vi "JPEG2000-Example.vi"() -> ()   [LabVIEW 2026]
uses:
  <vilib>/Utility/sysdir.llb/System Directory Type.ctl
panel:
  out "Image":T1(plugin-control)
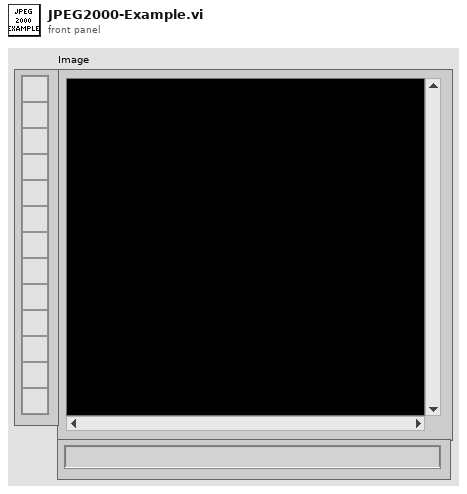
[diagram p1: front panel]
types:
  T1 = typedef "IMAQ Image.ctl" = refnum<image>
  T2 = typedef "System Directory Type.ctl" = i32
  T3 = typedef "Image Type" = u32
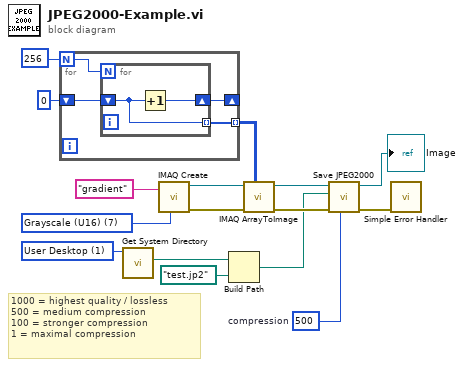
[diagram p0: block diagram]
diagram:
  w4 = T2 1 items=["User Home"=0, "User Desktop"=1, "User Documents"=2, "User Application Data"=3, "User Preferences"=4, "User Temporary"=5, "Public Documents"=6, "Public Application Data"=7, "Public Preferences"=8, "Public Cache"=13, "System Core Libraries"=9, "System Installed Libraries"=10, "Application Files"=11, "Boot Volume Root"=12] ("system directory type")
  w7 = 500  # compression
  w13 = T3 7 items=["Grayscale (U8)", "Grayscale (I16)", "Grayscale (SGL)", "Complex (CSG)", "RGB (U32)", "HSL (U32)", "RGB (U64)", "Grayscale (U16)"] ("Image Type")
  # "1000 = highest quality / lossless\n500 = medium compression\n100 = stronger compression\n1 = maximal compression"
  n1 = for {
    N: 256 -> [w20]
    shift-right: [w18] -> _
    shift-left: u16 0 -> [w19]
    tunnel: [w17] -> w11 mode=indexing
    n2 = for {
      N: w20 -> [_]
      shift-right: [w22] -> w18
      shift-left: w19 -> [w21]
      tunnel: [w21] -> w17 mode=indexing
      n3 = Increment(x=w21) -> (x+1=w22:u16)
    }
  }
  n4 = call <vilib>:"Get System Directory.vi"("system directory type"=w4) -> ("system directory"=w2:path)  [unwired: 10 in]
  n5 = call "IMAQ Create"("Image Name"="gradient", "Image Type"=w13) -> ("New Image"=w12:T1, "error out"=w5:errorcluster)  [unwired: 3 in]
  n6 = Build Path(base path=w2, name or relative path=path "test.jp2") -> (appended path=w1:path)
  n7 = call "IMAQ ArrayToImage"("Image Pixels (U16)"=w11, "error in (no error)"=w5, "Image"=w12) -> ("error out"=w9:errorcluster, "Image Out"=w10:T1)  [unwired: 7 in]
  n8 = call "Save JPEG2000.vi"("compression"=w7, "error in (no error)"=w9, "File Path"=w1, "Image in"=w10) -> ("error out"=w8:errorcluster, "Image out (dup)"=→"Image":T1)  [unwired: 6 in]
  n9 = call <vilib>:"Simple Error Handler.vi"("error in (no error)"=w8) -> ()  [unwired: 4 in, 5 out]
